vi "App_Query Data.vi"() -> ()   [LabVIEW 2015, in "Application 2.lvlib"]
uses:
  Application 2.lvlib
panel:
  out "Result":string caption="String"
  in  "Time List":i32(listbox)
  out "Electrocardiography":waveform(dbl)(graph) caption="Waveform Graph"
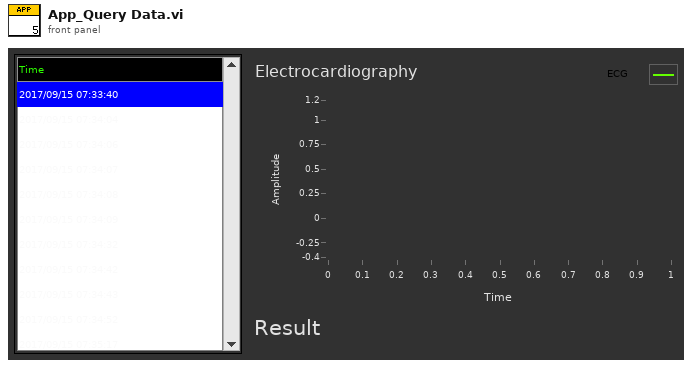
[diagram p1: front panel]
types:
  T1 = typedef "Data File Format.ctl" = cluster{"Data":waveform(dbl), "Abnormal?":bool, "Measure Time":timestamp, "User Name":string}
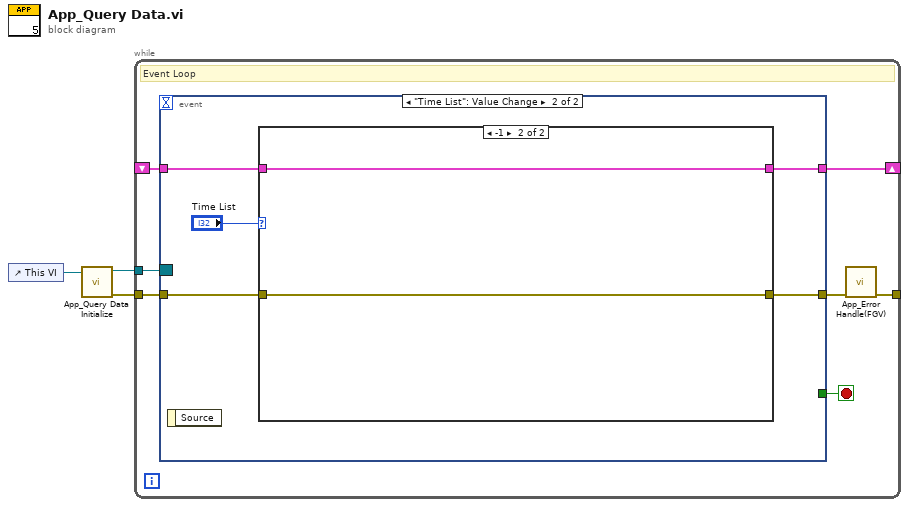
[diagram p0: block diagram]
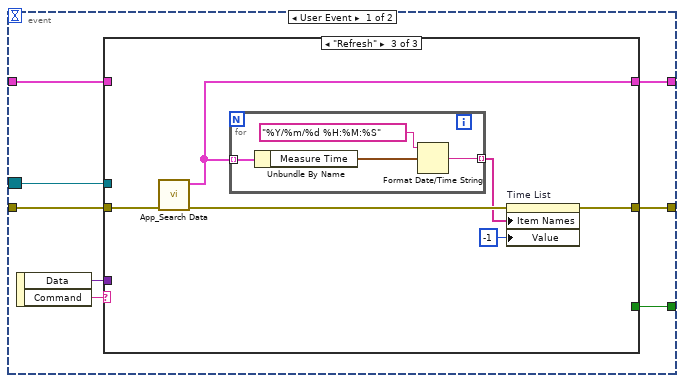
[diagram p2: hidden frame]
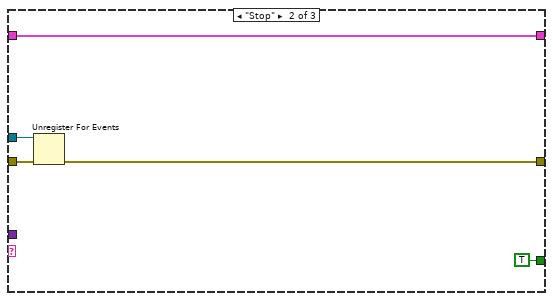
[diagram p4: hidden frame]
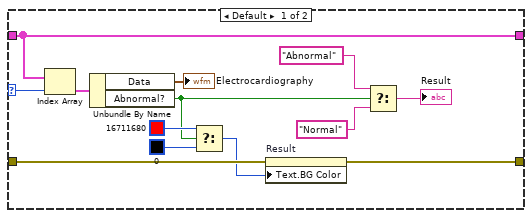
[diagram p5: hidden frame]
diagram:
  n1 = control-ref of="This VI"() -> (w3:refnum<vi>)
  n2 = call "App_Query Data Initialize.vi"("VI Reference"=w3) -> ("error out"=w1:errorcluster, "Event Registration Refnum"=w2:refnum<event-registration>)  [unwired: 9 in]
  n3 = while {
    tunnel: w2 -> [w10]
    tunnel: w1 -> [w9]
    tunnel: [w7] -> _
    shift-right: [w5] -> _
    shift-left: _ -> [w4]
    stop <- w6 stop-if-true
    # "Event Loop"
    n4 = event shown="[1] \"Time List\": Value Change" {
      selector: w10 -> [w15 _]
      dyn-events: _ -> [_ _]
      timeout: _ -> [_ _]
      tunnel: w9 -> [w16 w37]
      tunnel: [w14 w36] -> w8
      tunnel: [w13 _] -> w6
      tunnel: [w12 w38] -> w5
      tunnel: w4 -> [w11 w39]
      event User Event {
        n5 = event-data() -> ("Data"=w17:variant, "Command"=w18:string)  [unwired: 1 in]
        n6 = case shown="\"Refresh\"" w18 {
          tunnel: w17 -> [_ _ _]
          tunnel: w16 -> [w20 w25 w31]
          tunnel: w15 -> [_ w24 _]
          tunnel: [w20 w23 w27] -> w14
          tunnel: [_ TRUE _] -> w13
          tunnel: [w19 w21 w30] -> w12
          tunnel: w11 -> [w19 w21 _]
          frame Default {
          }
          frame "Stop" {
            n7 = Unregister For Events(event registration refnum=w24, error in=w25) -> (error out=w23:errorcluster)
          }
          frame "Refresh" {
            n8 = call "App_Search Data.vi"("error in"=w31) -> ("error out"=w29:errorcluster, "Log Data"=w30:T1[])  [unwired: 9 in]
            n9 = for {
              tunnel: w30 -> [w35] mode=indexing
              tunnel: [w32] -> w28 mode=indexing
              n10 = Unbundle By Name(w35) -> ("Measure Time"=w33:timestamp)
              n11 = Format Date/Time String(time format string (%c)="%Y/%m/%d %H:%M:%S", seconds (now)=w33) -> (date/time string=w32:string)  [unwired: 1 in]
            }
            n12 = property on="Time List" class="LstBox (strict)"(error in=w29, "Item Names"=w28, "Value"=-1 ("Time List")) -> (error out=w27:errorcluster)  [unwired: 1 in, 1 out]
          }
        }
      }
      event "Time List": Value Change {
        n13 = event-data() -> ()  [unwired: 1 in, 1 out]
        n14 = case shown="-1" "Time List" {
          selector: "Time List" -> [w53 _]
          tunnel: w39 -> [w50 w55]
          tunnel: [w50 w55] -> w38
          tunnel: w37 -> [w49 w54]
          tunnel: [w44 w54] -> w36
          frame Default {
            n15 = Index Array(array=w50, index=w53) -> (element=w52:T1)
            n16 = Unbundle By Name(w52) -> ("Data"=→"Electrocardiography":waveform(dbl), "Abnormal?"=w45:bool)
            n17 = Select(t=u32 16711680, s=w45, f=u32 0) -> (s? t:f=w46:u32)
            n18 = property on="Result" class="Str"(error in=w49, "Text.BG Color"=w46) -> (error out=w44:errorcluster)  [unwired: 1 in, 1 out]
            n19 = Select(t="Abnormal", s=w45, f="Normal") -> (s? t:f=→"Result":string)
          }
          frame -1 {
          }
        }
      }
    }
    n20 = call "App_Error Handle(FGV).vi"("error in"=w8) -> ("error out"=w7:errorcluster)  [unwired: 9 in, 1 out]
  }
